vi "merFISH_select_laser_line.vi"(3 "Laser line":i32, 4 "Total number of lines":i32, 5 "Laser array":T2(array[cluster])) -> (0 "Next laser line":i32, 2 "excitation cluster":T1)   [LabVIEW 2015]
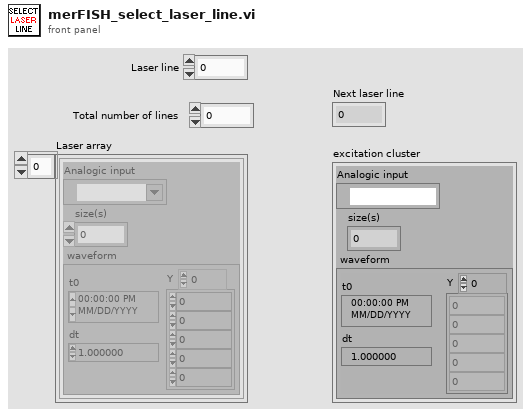
[diagram p1: front panel]
types:
  T1 = cluster{"Analogic input":tag, "size(s)":i32, " waveform":waveform(dbl)}
  T2 = cluster{"Analogic input":tag, "size(s)":i32, " waveform":waveform(dbl)}[]
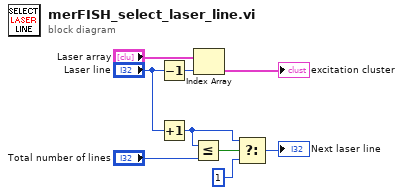
[diagram p0: block diagram]
diagram:
  n1 = Decrement(x="Laser line") -> (x-1=w2:i32)
  n2 = Increment(x="Laser line") -> (x+1=w3:i32)
  n3 = Less Or Equal?(x=w3, y="Total number of lines") -> (x <= y?=w5:bool)
  n4 = Index Array(array="Laser array", index=w2) -> (element=→"excitation cluster":T1)
  n5 = Select(t=w3, s=w5, f=1 ("t")) -> (s? t:f=→"Next laser line":i32)
